vi "Read Animal.vi"(8 "error in (no error)":errorcluster, 11 "Animal Test In":refnum<class "Animal Test.lvclass">) -> (0 "error out":errorcluster, 2 "Animal.lvclass":refnum<class "Animal.lvclass">, 3 "Animal Test Out":refnum<class "Animal Test.lvclass">)   [LabVIEW 2020, in "Animal Test.lvclass"]
doc: "Read Animal"
uses:
  Animal Test.lvclass
  Animal Classes/Animal/Animal.lvclass
  Animal Test.lvclass/Animal Test.ctl
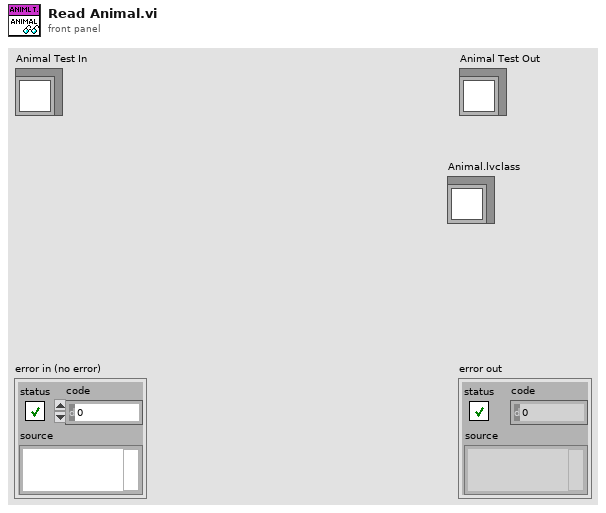
[diagram p1: front panel]
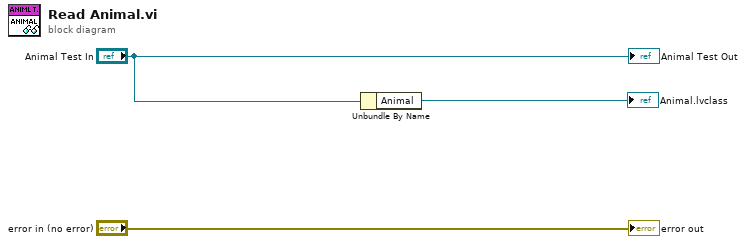
[diagram p0: block diagram]
diagram:
  n1 = Unbundle By Name("Animal Test In") -> ("Animal"=→"Animal.lvclass":refnum<class "Animal.lvclass">)
  "error out" <- "error in (no error)"
  "Animal Test Out" <- "Animal Test In"
